vi "多个参数加标回收启动器.vi"(10 "流程":T1, 11 "启用参数选择":T2) -> ()   [LabVIEW 2016, in "质控单元V4.lvlib"]
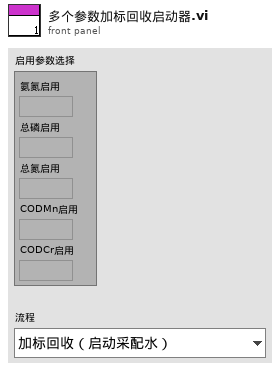
[diagram p1: front panel]
types:
  T1 = typedef "质控单元V4.lvlib/测试流程.ctl" = enum16{"加标回收（启动采配水）", "加标回收（不启动采配水）", "水样测试（启动采配水）", "水样测试（不启动采配水）", "平行样测试（启动采配水）", "平行样测试（不启动采配水）", "集成干预测试"}
  T2 = cluster{"氨氮启用":bool, "总磷启用":bool, "总氮启用":bool, "CODMn启用":bool, "CODCr启用":bool}
  T3 = typedef "质控单元V4.lvlib/测试子流程.ctl" = enum16{"水样测试（润洗采样分开）", "水样测试（润洗采样合并）", "水样测试（不启动采配水）", "加标回收（润洗采样分开）", "加标回收（润洗采样合并）", "加标回收（不启动采配水）", "集成干预测试", "平行样测试", "平行样测试（不启动采配水）"}
  T4 = cluster{"氨氮":bool, "总磷":bool, "总氮":bool, "CODMn":bool, "CODCr":bool}
  T5 = typedef "质控单元V4.lvlib/质控slave id.ctl" = enum16{"null", "氨氮", "总磷", "总氮", "CODMn", "CODCr"}
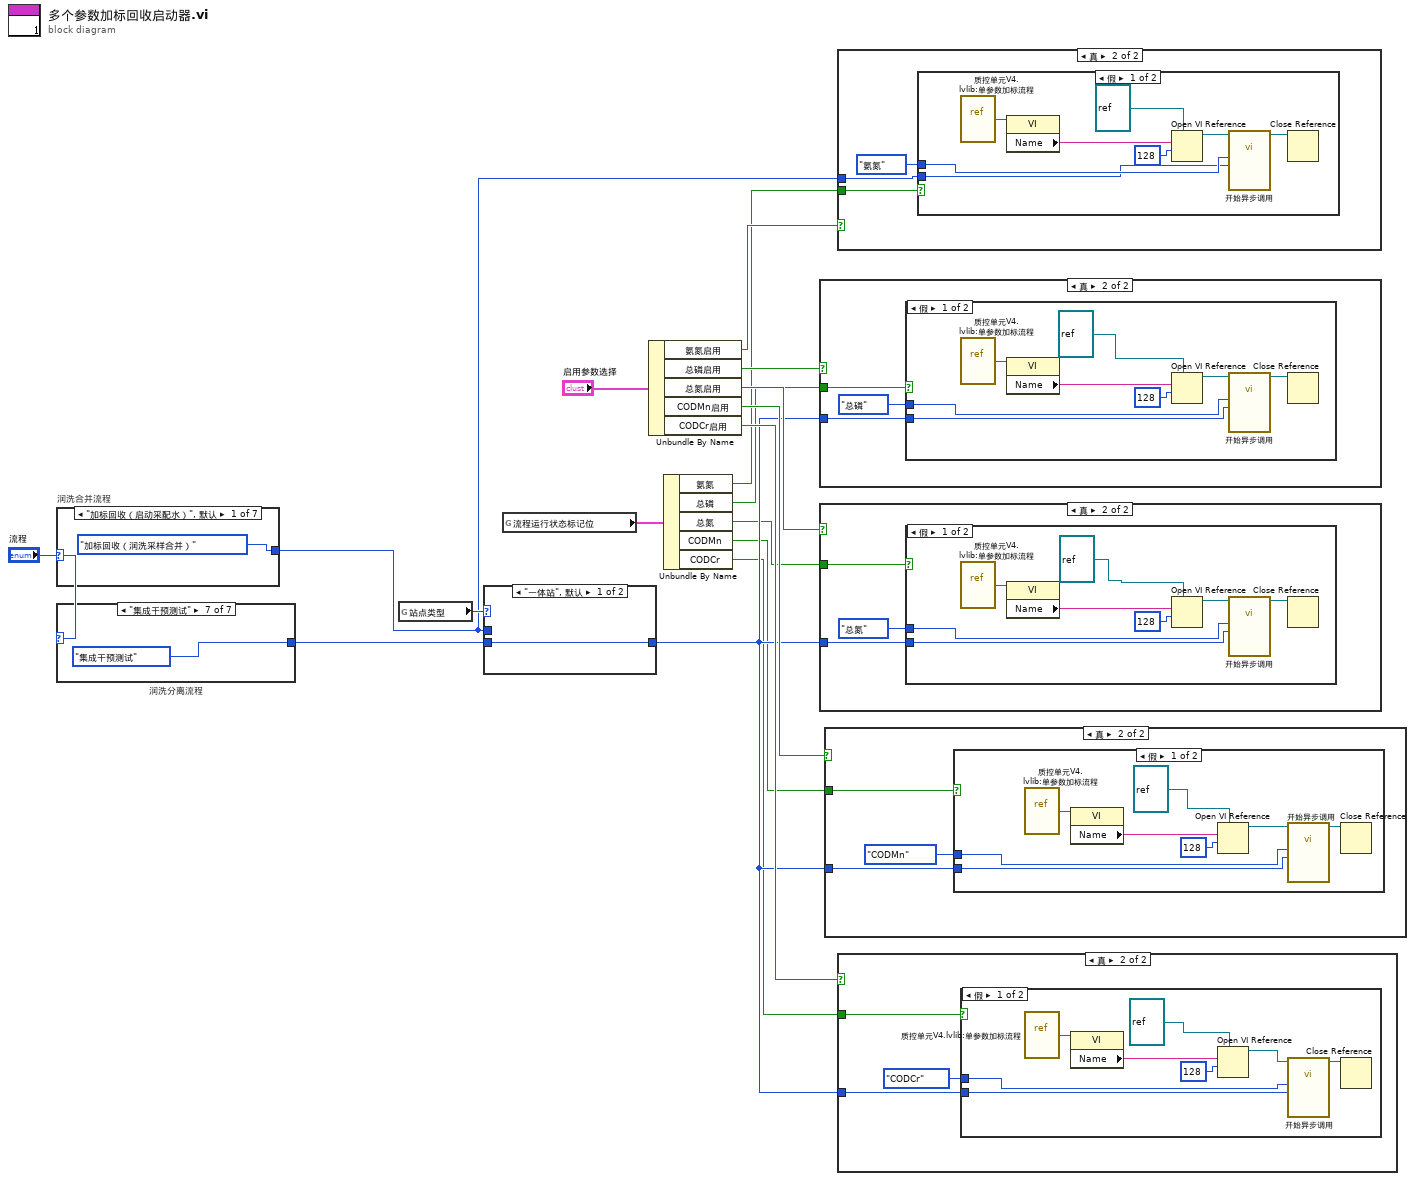
[diagram p0: block diagram]
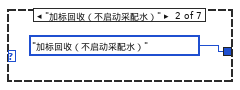
[diagram p2: hidden frame]
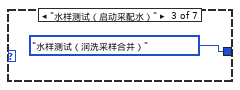
[diagram p3: hidden frame]
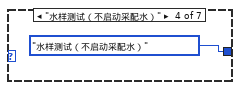
[diagram p4: hidden frame]
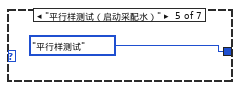
[diagram p5: hidden frame]
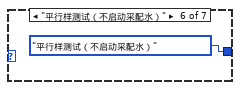
[diagram p6: hidden frame]
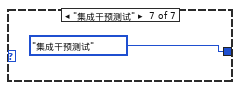
[diagram p7: hidden frame]
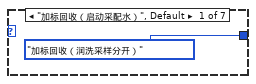
[diagram p8: hidden frame]
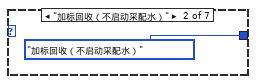
[diagram p9: hidden frame]
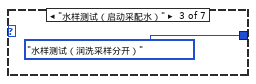
[diagram p10: hidden frame]
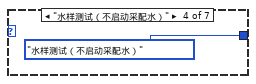
[diagram p11: hidden frame]
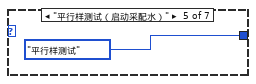
[diagram p12: hidden frame]
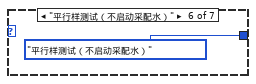
[diagram p13: hidden frame]
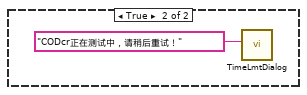
[diagram p16: hidden frame]
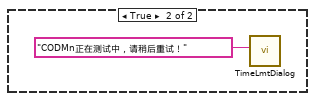
[diagram p18: hidden frame]
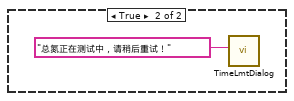
[diagram p20: hidden frame]
diagram:
  n1 = case "润洗合并流程" shown="\"加标回收（启动采配水）\", 默认" "流程" {
    tunnel: [测试子流程."加标回收（润洗采样合并）" ("流程类型") 测试子流程."加标回收（不启动采配水）" ("流程类型") 测试子流程."水样测试（润洗采样合并）" ("流程类型") 测试子流程."水样测试（不启动采配水）" ("流程类型") 测试子流程."平行样测试" ("流程类型") 测试子流程."平行样测试（不启动采配水）" ("流程类型") 测试子流程."集成干预测试" ("流程类型")] -> w8
    frame "加标回收（启动采配水）", Default {
    }
    frame "加标回收（不启动采配水）" {
    }
    frame "水样测试（启动采配水）" {
    }
    frame "水样测试（不启动采配水）" {
    }
    frame "平行样测试（启动采配水）" {
    }
    frame "平行样测试（不启动采配水）" {
    }
    frame "集成干预测试" {
    }
  }
  n2 = case "润洗分离流程" shown="\"集成干预测试\"" "流程" {
    tunnel: [测试子流程."加标回收（润洗采样分开）" ("流程类型") 测试子流程."加标回收（不启动采配水）" ("流程类型") 测试子流程."水样测试（润洗采样分开）" ("流程类型") 测试子流程."水样测试（不启动采配水）" ("流程类型") 测试子流程."平行样测试" ("流程类型") 测试子流程."平行样测试（不启动采配水）" ("流程类型") 测试子流程."集成干预测试" ("流程类型")] -> w9
    frame "加标回收（启动采配水）", Default {
    }
    frame "加标回收（不启动采配水）" {
    }
    frame "水样测试（启动采配水）" {
    }
    frame "水样测试（不启动采配水）" {
    }
    frame "平行样测试（启动采配水）" {
    }
    frame "平行样测试（不启动采配水）" {
    }
    frame "集成干预测试" {
    }
  }
  n3 = global read "系统交互.vi" "站点类型"() -> (w11:enum16{"一体站", "固定站", "浮船"})
  n4 = case shown="\"一体站\", 默认" w11 {
    tunnel: w9 -> [w32 _]
    tunnel: w8 -> [_ w33]
    tunnel: [w32 w33] -> w7
    frame "一体站", Default {
    }
    frame "固定站" {
    }
  }
  n5 = global read "ZK非断电保存全局变量.vi" "流程运行状态标记位"() -> (w6:T4)
  n6 = Unbundle By Name("启用参数选择") -> ("氨氮启用"=w16:bool, "总磷启用"=w15:bool, "总氮启用"=w14:bool, "CODMn启用"=w13:bool, "CODCr启用"=w12:bool)
  n7 = Unbundle By Name(w6) -> ("氨氮"=w5:bool, "总磷"=w4:bool, "总氮"=w3:bool, "CODMn"=w2:bool, "CODCr"=w1:bool)
  n8 = case shown="真" w15 {
    tunnel: w7 -> [_ w35]
    tunnel: w4 -> [_ w34]
    frame False {
    }
    frame True {
      n9 = case shown="假" w34 {
        tunnel: w35 -> [w39 _]
        tunnel: 质控slave_id."总磷" ("Slave ID") -> [w38 _]
        frame False {
          n10 = vi-ref "质控单元V4.lvlib:单参数加标流程.vi"() -> (w40:refnum<vi>)
          n11 = property class="VI"(reference=w40) -> ("Name"=w41:string)  [unwired: 1 in, 2 out]
          n12 = Open VI Reference(type specifier VI Refnum (for type only)=refnum<vi> refnum, vi path=w41, options=128 ("选项")) -> (vi reference=w43:refnum<vi>)  [unwired: 3 in, 1 out]
          n13 = call-by-ref "开始异步调用"(reference=w43, "流程类型"=w39, "Slave ID"=w38) -> (reference out=w44:refnum<vi>)  [unwired: 11 in, 1 out]
          n14 = Close Reference(reference=w44) -> ()  [unwired: 1 in, 1 out]
        }
        frame True {
          n15 = call "TimeLmtDialog.vi"("Infoin"="总磷正在测试中，请稍后重试！" ("消息")) -> ()  [unwired: 11 in]
        }
      }
    }
  }
  n16 = case shown="真" w14 {
    tunnel: w7 -> [_ w47]
    tunnel: w3 -> [_ w46]
    frame False {
    }
    frame True {
      n17 = case shown="假" w46 {
        tunnel: w47 -> [w50 _]
        tunnel: 质控slave_id."总氮" ("Slave ID") -> [w51 _]
        frame False {
          n18 = vi-ref "质控单元V4.lvlib:单参数加标流程.vi"() -> (w52:refnum<vi>)
          n19 = property class="VI"(reference=w52) -> ("Name"=w53:string)  [unwired: 1 in, 2 out]
          n20 = Open VI Reference(type specifier VI Refnum (for type only)=refnum<vi> refnum, vi path=w53, options=128 ("选项")) -> (vi reference=w55:refnum<vi>)  [unwired: 3 in, 1 out]
          n21 = call-by-ref "开始异步调用"(reference=w55, "流程类型"=w50, "Slave ID"=w51) -> (reference out=w56:refnum<vi>)  [unwired: 11 in, 1 out]
          n22 = Close Reference(reference=w56) -> ()  [unwired: 1 in, 1 out]
        }
        frame True {
          n23 = call "TimeLmtDialog.vi"("Infoin"="总氮正在测试中，请稍后重试！" ("消息")) -> ()  [unwired: 11 in]
        }
      }
    }
  }
  n24 = case shown="真" w13 {
    tunnel: w7 -> [_ w58]
    tunnel: w2 -> [_ w59]
    frame False {
    }
    frame True {
      n25 = case shown="假" w59 {
        tunnel: w58 -> [w63 _]
        tunnel: 质控slave_id."CODMn" ("Slave ID") -> [w62 _]
        frame False {
          n26 = vi-ref "质控单元V4.lvlib:单参数加标流程.vi"() -> (w64:refnum<vi>)
          n27 = property class="VI"(reference=w64) -> ("Name"=w65:string)  [unwired: 1 in, 2 out]
          n28 = Open VI Reference(type specifier VI Refnum (for type only)=refnum<vi> refnum, vi path=w65, options=128 ("选项")) -> (vi reference=w67:refnum<vi>)  [unwired: 3 in, 1 out]
          n29 = call-by-ref "开始异步调用"(reference=w67, "流程类型"=w63, "Slave ID"=w62) -> (reference out=w68:refnum<vi>)  [unwired: 11 in, 1 out]
          n30 = Close Reference(reference=w68) -> ()  [unwired: 1 in, 1 out]
        }
        frame True {
          n31 = call "TimeLmtDialog.vi"("Infoin"="CODMn正在测试中，请稍后重试！" ("消息")) -> ()  [unwired: 11 in]
        }
      }
    }
  }
  n32 = case shown="真" w16 {
    tunnel: w8 -> [_ w72]
    tunnel: w5 -> [_ w71]
    frame False {
    }
    frame True {
      n33 = case shown="假" w71 {
        tunnel: w72 -> [w74 _]
        tunnel: 质控slave_id."氨氮" ("Slave ID") -> [w75 _]
        frame False {
          n34 = vi-ref "质控单元V4.lvlib:单参数加标流程.vi"() -> (w76:refnum<vi>)
          n35 = property class="VI"(reference=w76) -> ("Name"=w77:string)  [unwired: 1 in, 2 out]
          n36 = Open VI Reference(type specifier VI Refnum (for type only)=refnum<vi> refnum, vi path=w77, options=128 ("选项")) -> (vi reference=w79:refnum<vi>)  [unwired: 3 in, 1 out]
          n37 = call-by-ref "开始异步调用"(reference=w79, "流程类型"=w74, "Slave ID"=w75) -> (reference out=w80:refnum<vi>)  [unwired: 11 in, 1 out]
          n38 = Close Reference(reference=w80) -> ()  [unwired: 1 in, 1 out]
        }
        frame True {
          n39 = call "TimeLmtDialog.vi"("Infoin"="氨氮正在测试中，请稍后重试！" ("消息")) -> ()  [unwired: 11 in]
        }
      }
    }
  }
  n40 = case shown="真" w12 {
    tunnel: w7 -> [_ w82]
    tunnel: w1 -> [_ w83]
    frame False {
    }
    frame True {
      n41 = case shown="假" w83 {
        tunnel: w82 -> [w86 _]
        tunnel: 质控slave_id."CODCr" ("Slave ID") -> [w87 _]
        frame False {
          n42 = vi-ref "质控单元V4.lvlib:单参数加标流程.vi"() -> (w88:refnum<vi>)
          n43 = property class="VI"(reference=w88) -> ("Name"=w89:string)  [unwired: 1 in, 2 out]
          n44 = Open VI Reference(type specifier VI Refnum (for type only)=refnum<vi> refnum, vi path=w89, options=128 ("选项")) -> (vi reference=w91:refnum<vi>)  [unwired: 3 in, 1 out]
          n45 = call-by-ref "开始异步调用"(reference=w91, "流程类型"=w86, "Slave ID"=w87) -> (reference out=w92:refnum<vi>)  [unwired: 11 in, 1 out]
          n46 = Close Reference(reference=w92) -> ()  [unwired: 1 in, 1 out]
        }
        frame True {
          n47 = call "TimeLmtDialog.vi"("Infoin"="CODcr正在测试中，请稍后重试！" ("消息")) -> ()  [unwired: 11 in]
        }
      }
    }
  }
